vi "Read Sender Enqueuer ID string.vi"(8 "error in (no error)":errorcluster, 11 "Publisher Msg in":refnum<class "Publisher Msg.lvclass">) -> (0 "error out":errorcluster, 2 "Sender Enqueuer ID string":string, 3 "Publisher Msg out":refnum<class "Publisher Msg.lvclass">)   [LabVIEW 2020, in "Publisher.lvlib" / "Publisher Msg.lvclass"]
doc: "Read the Enqueuer ID String of the sending actor."
uses:
  Publisher Msg.lvclass
  Publisher Msg.lvclass/Publisher Msg.ctl
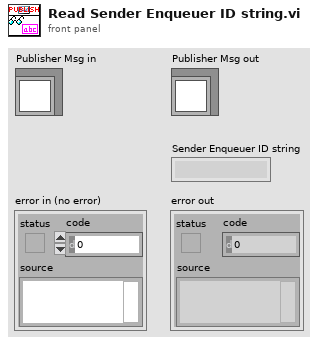
[diagram p1: front panel]
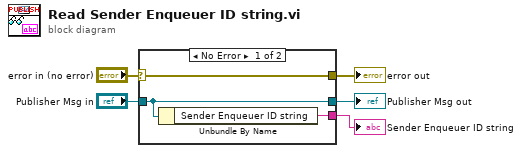
[diagram p0: block diagram]
diagram:
  n1 = case shown="No Error" "error in (no error)" {
    selector: "error in (no error)" -> [w8 w9]
    tunnel: [w8 w9] -> w4
    tunnel: [w7 w10] -> w2
    tunnel: "Publisher Msg in" -> [w7 w10]
    tunnel: [w6 _] -> w1
    frame No Error {
      n2 = Unbundle By Name(w7) -> ("Sender Enqueuer ID string"=w6:string)
    }
    frame Error {
    }
  }
  "error out" <- w4
  "Publisher Msg out" <- w2
  "Sender Enqueuer ID string" <- w1
